vi "Read FPGA VI Reference Out.vi"(8 "error in (no error)":errorcluster, 11 "FpgaRunner in":refnum<class "FpgaRunner.lvclass">) -> (0 "error out":errorcluster, 2 "FPGA VI Reference Out":refnum<k20>, 3 "FpgaRunner out":refnum<class "FpgaRunner.lvclass">)   [LabVIEW 2020, in "FpgaRunner.lvclass"]
uses:
  FpgaRunner.lvclass
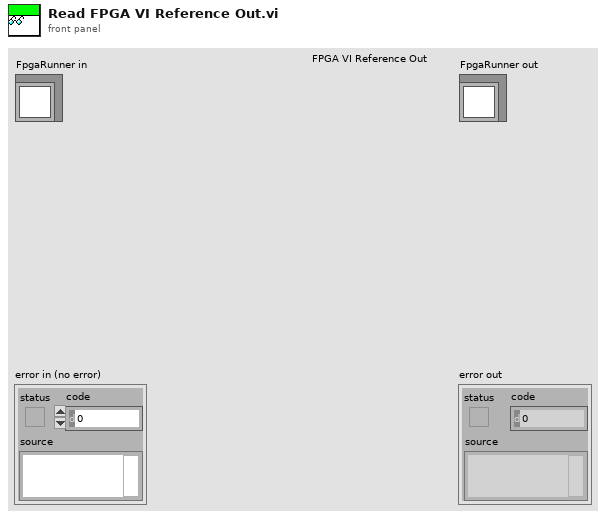
[diagram p1: front panel]
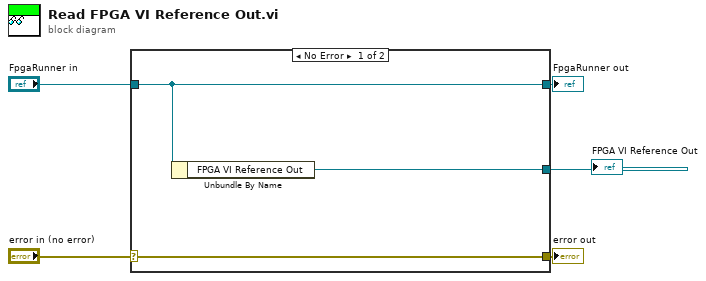
[diagram p0: block diagram]
diagram:
  n1 = case shown="No Error" "error in (no error)" {
    selector: "error in (no error)" -> [w8 w9]
    tunnel: [w8 w9] -> w4
    tunnel: [w7 w10] -> w2
    tunnel: "FpgaRunner in" -> [w7 w10]
    tunnel: [w6 _] -> w1
    frame No Error {
      n2 = Unbundle By Name(w7) -> ("FPGA VI Reference Out"=w6:refnum<k20>)
    }
    frame Error {
    }
  }
  "error out" <- w4
  "FpgaRunner out" <- w2
  "FPGA VI Reference Out" <- w1
